vi "Get Disable Symbol Value.vi"(8 "error in (no error)":errorcluster, 10 "Disable Symbol":string, 11 "TargetItem Refnum":refnum<vi>) -> (0 "error out":errorcluster, 1 "Found?":bool, 2 "Value":string, 3 "Duplicated TargetItem Refnum":refnum<vi>)   [LabVIEW 2021, in "Personality.lvlib"]
doc: "Gets the specified disable symbol value from specified target item reference."
uses:
  <vilib>/myRIO/Common/FPGA Personality Framework/Personality.lvlib
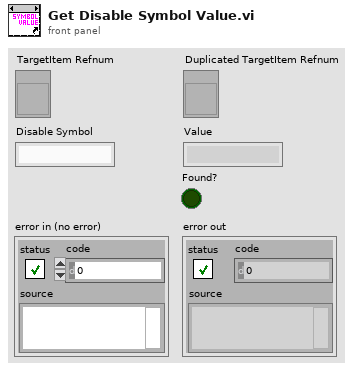
[diagram p1: front panel]
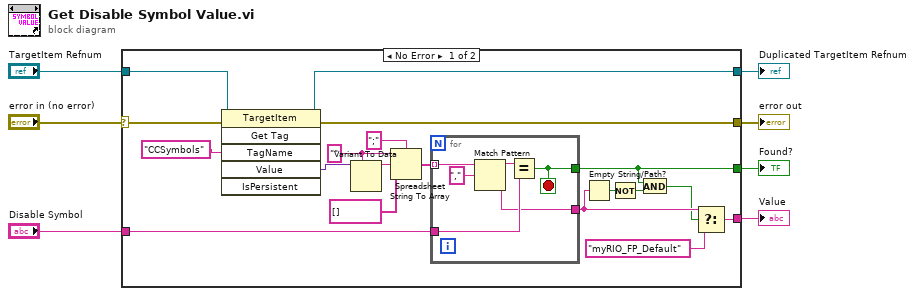
[diagram p0: block diagram]
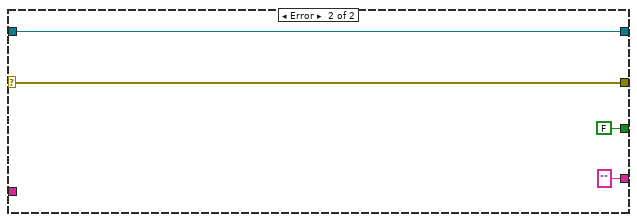
[diagram p2: hidden frame]
diagram:
  n1 = case shown="No Error" "error in (no error)" {
    selector: "error in (no error)" -> [w24 w36]
    tunnel: [w26 w36] -> w7
    tunnel: "Disable Symbol" -> [w25 _]
    tunnel: [w9 FALSE] -> w4
    tunnel: [w15 "" ("f")] -> w3
    tunnel: "TargetItem Refnum" -> [w14 w33]
    tunnel: [w13 w33] -> w1
    frame No Error {
      w17 = "" ("format string")
      n2 = invoke class="TargetItem" method="Get Tag"(reference=w14, error in=w24, "TagName"="CCSymbols" ("Tag Name")) -> (reference out=w13:refnum<vi>, error out=w26:errorcluster, "Value"=w23:variant)  [unwired: 3 in, 3 out]
      n3 = Variant To Data(type=w17, Variant=w23) -> (data=w21:string)  [unwired: 1 in, 1 out]
      n4 = Spreadsheet String To Array(delimiter (Tab)=";", format string=w17, spreadsheet string=w21, array type (2D Dbl)=string[] []) -> (array=w18:string[])
      n5 = for {
        tunnel: w18 -> [w31] mode=indexing
        tunnel: w25 -> [w29]
        tunnel: [w28] -> w9
        tunnel: [w27] -> w10
        stop <- w28 stop-if-true
        n6 = Match Pattern(string=w31, regular expression=",") -> (before substring=w30:string, after substring=w27:string)  [unwired: 1 in, 2 out]
        n7 = Equal?(x=w30, y=w29) -> (x = y?=w28:bool)
      }
      n8 = Empty String/Path?(string/path=w10) -> (empty?=w11:bool)
      n9 = Not(x=w11) -> (.not. x?=w12:bool)
      n10 = And(x=w9, y=w12) -> (x .and. y?=w8:bool)
      n11 = Select(t=w10, s=w8, f="myRIO_FP_Default") -> (s? t:f=w15:string)
    }
    frame Error {
    }
  }
  "Value" <- w3
  "error out" <- w7
  "Found?" <- w4
  "Duplicated TargetItem Refnum" <- w1
